vi "microFPGA_laser_duration_addr_10_ctrl.vi"(0 "VISA resource name":refnum<visa-resource-name>, 1 "laser channel":u16(ring)=3 items=["channel No 0", "channel No 1", "channel No 2", "channel No 3", "channel No 4", "channel No 5", "channel No 6"], 2 "write or read":u16(ring) items=["read", "write"], 5 "duration write":u32(slide) max=65535 step=1 scale=0.0..65535.0 scale format="%u us", 11 "error in (no error)":errorcluster) -> (4 "VISA resource name 2":refnum<visa-resource-name>, 6 "duration read":u32(slide) max=65535 step=1 scale=0.0..65535.0 scale format="%u us", 8 "value write confirm":bool, 10 "abort_wrong_input":bool, 15 "error out":errorcluster)   [LabVIEW 2018]
panel:
  out "mode read string answer":string
  out "mode read string":string
  out "mode write string":string
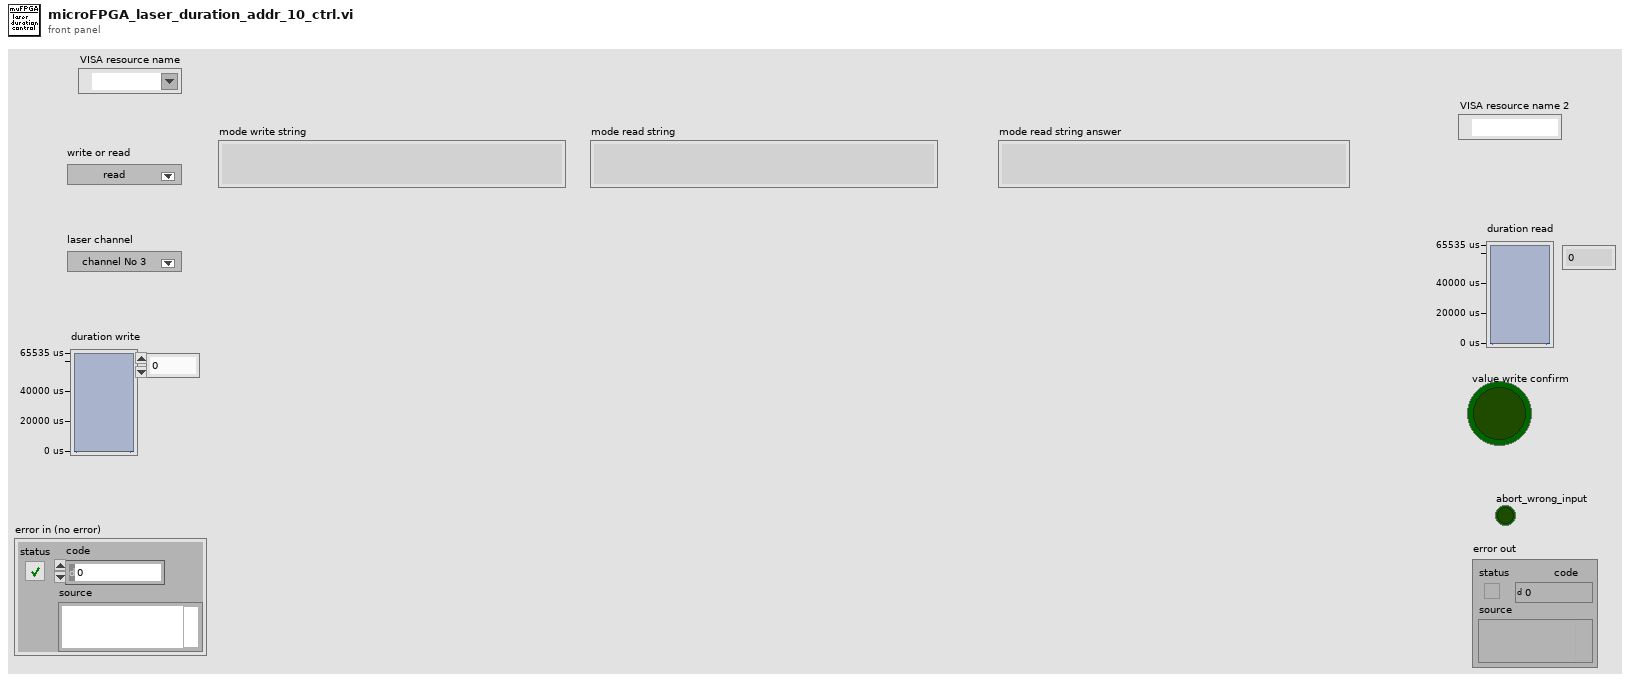
[diagram p1: front panel]
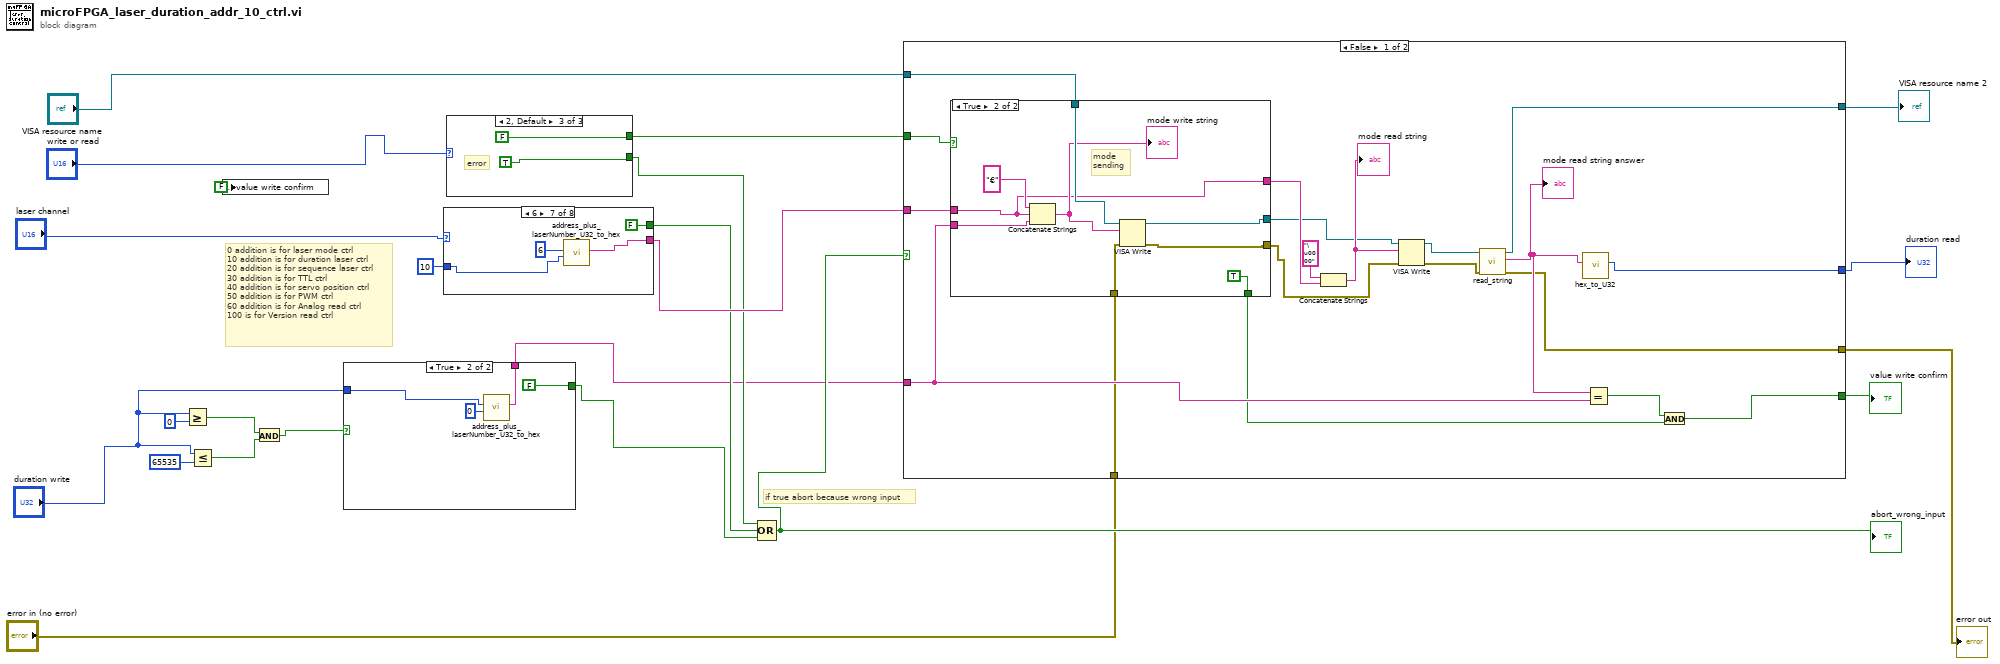
[diagram p0: block diagram]
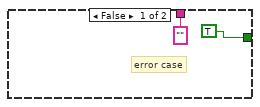
[diagram p2: hidden frame]
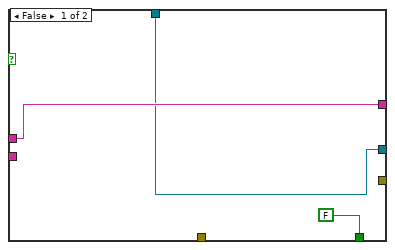
[diagram p3: hidden frame]
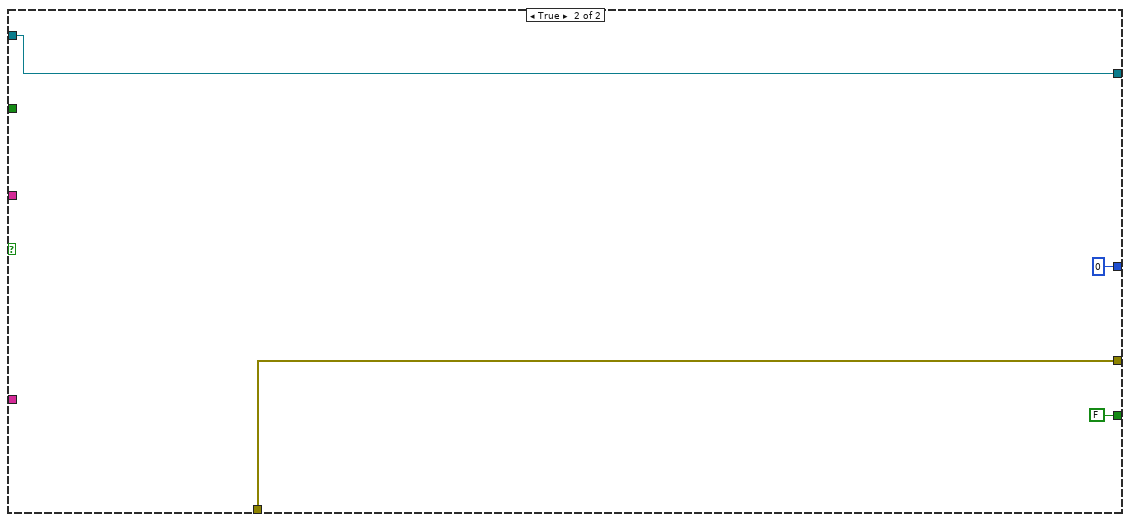
[diagram p4: hidden frame]
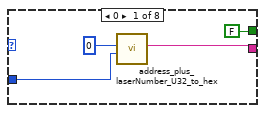
[diagram p5: hidden frame]
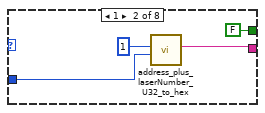
[diagram p6: hidden frame]
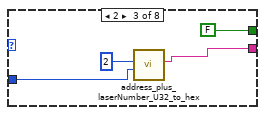
[diagram p7: hidden frame]
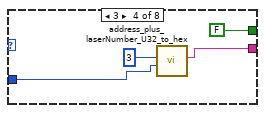
[diagram p8: hidden frame]
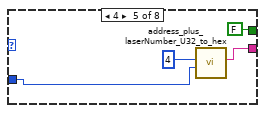
[diagram p9: hidden frame]
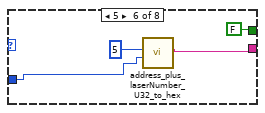
[diagram p10: hidden frame]
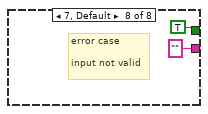
[diagram p11: hidden frame]
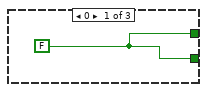
[diagram p12: hidden frame]
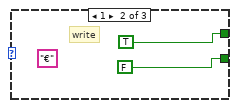
[diagram p13: hidden frame]
diagram:
  # "0 addition is for laser mode ctrl\n10 addition is for duration laser ctrl\n20 addition is for sequence laser ctrl\n30 addition is for TTL ctrl\n40 addition is for servo position ctrl\n50 addition is for PWM ctrl\n60 addition is for Analog read ctrl\n100 is for Version read ctrl"
  # "if true abort because wrong input"
  n1 = Greater Or Equal?(x="duration write", y=u32 0) -> (x >= y?=w7:bool)
  n2 = Less Or Equal?(x="duration write", y=u32 65535) -> (x <= y?=w6:bool)
  n3 = local write "value write confirm"(FALSE ("value confirm")) -> ()
  n4 = And(x=w7, y=w6) -> (x .and. y?=w5:bool)
  n5 = case shown="True" w5 {
    tunnel: "duration write" -> [_ w28]
    tunnel: [TRUE FALSE] -> w4
    tunnel: ["" ("string 5") w26] -> w3
    frame False {
      # "error case"
    }
    frame True {
      n6 = call "address_plus_laserNumber_U32_to_hex.vi"("adress offset"=u32 0, "y 3"=w28) -> ("string 5"=w26:string)  [unwired: 8 in]
    }
  }
  n7 = case shown="6" "laser channel" {
    tunnel: [w31 w35 w39 w43 w47 w51 w55 "" ("string 5")] -> w21
    tunnel: [FALSE FALSE FALSE FALSE FALSE FALSE FALSE TRUE] -> w17
    tunnel: u32 10 ("adress offset") -> [w30 w34 w38 w42 w46 w50 w54 _]
    frame 0 {
      n8 = call "address_plus_laserNumber_U32_to_hex.vi"("adress offset"=w30, "y 3"=u32 0) -> ("string 5"=w31:string)  [unwired: 8 in]
    }
    frame 1 {
      n9 = call "address_plus_laserNumber_U32_to_hex.vi"("adress offset"=w34, "y 3"=u32 1) -> ("string 5"=w35:string)  [unwired: 8 in]
    }
    frame 2 {
      n10 = call "address_plus_laserNumber_U32_to_hex.vi"("adress offset"=w38, "y 3"=u32 2) -> ("string 5"=w39:string)  [unwired: 8 in]
    }
    frame 3 {
      n11 = call "address_plus_laserNumber_U32_to_hex.vi"("adress offset"=w42, "y 3"=u32 3) -> ("string 5"=w43:string)  [unwired: 8 in]
    }
    frame 4 {
      n12 = call "address_plus_laserNumber_U32_to_hex.vi"("adress offset"=w46, "y 3"=u32 4) -> ("string 5"=w47:string)  [unwired: 8 in]
    }
    frame 5 {
      n13 = call "address_plus_laserNumber_U32_to_hex.vi"("adress offset"=w50, "y 3"=u32 5) -> ("string 5"=w51:string)  [unwired: 8 in]
    }
    frame 6 {
      n14 = call "address_plus_laserNumber_U32_to_hex.vi"("adress offset"=w54, "y 3"=u32 6) -> ("string 5"=w55:string)  [unwired: 8 in]
    }
    frame 7, Default {
      # "error case\n\ninput not valid"
    }
  }
  n15 = case shown="2, Default" "write or read" {
    tunnel: [w60 TRUE FALSE] -> w20
    tunnel: [w60 FALSE TRUE] -> w18
    frame 0 {
      w60 = FALSE
    }
    frame 1 {
      (unwired) "€" ("hex")
      # "write"
    }
    frame 2, Default {
      # "error"
    }
  }
  n16 = Compound Arithmetic op=OR(w18, w17, w4) -> (w15:bool)
  "abort_wrong_input" <- w15
  n17 = case shown="False" w15 {
    tunnel: "VISA resource name" -> [w83 w97]
    tunnel: w21 -> [w80 _]
    tunnel: w20 -> [w74 _]
    tunnel: w3 -> [w72 _]
    tunnel: [w71 u32 0 ("U32")] -> w1
    tunnel: [w65 FALSE] -> w16
    tunnel: [w70 w97] -> w14
    tunnel: "error in (no error)" -> [w69 w96]
    tunnel: [w68 w96] -> w12
    frame False {
      n18 = case shown="True" w74 {
        tunnel: w80 -> [w86 w92]
        tunnel: w83 -> [w85 w94]
        tunnel: [w86 w92] -> w81
        tunnel: w72 -> [_ w91]
        tunnel: [w85 w90] -> w76
        tunnel: [_ w89] -> w75
        tunnel: w69 -> [_ w88]
        tunnel: [FALSE TRUE] -> w67
        frame False {
        }
        frame True {
          # "mode \nsending"
          n19 = Concatenate Strings("€" ("string"), w92, w91) -> (w93:string)
          "mode write string" <- w93
          n20 = VISA Write(VISA resource name=w94, write buffer=w93, error in (no error)=w88) -> (VISA resource name out=w90:refnum<visa-resource-name>, error out=w89:errorcluster)  [unwired: 1 out]
        }
      }
      n21 = Concatenate Strings("\u0000" ("string"), w81) -> (w79:string)
      "mode read string" <- w79
      n22 = VISA Write(VISA resource name=w76, write buffer=w79, error in (no error)=w75) -> (VISA resource name out=w78:refnum<visa-resource-name>, error out=w77:errorcluster)  [unwired: 1 out]
      n23 = call "read_string.vi"("error in (no error)"=w77, "VISA resource name 2"=w78) -> ("error out"=w68:errorcluster, "read buffer"=w73:string, "VISA resource name"=w70:refnum<visa-resource-name>)  [unwired: 7 in]
      "mode read string answer" <- w73
      n24 = call "hex_to_U32.vi"("hex"=w73) -> ("U32"=w71:u32)  [unwired: 9 in]
      n25 = Equal?(x=w73, y=w72) -> (x = y?=w66:bool)
      n26 = And(x=w66, y=w67) -> (x .and. y?=w65:bool)
    }
    frame True {
    }
  }
  "value write confirm" <- w16
  "VISA resource name 2" <- w14
  "error out" <- w12
  "duration read" <- w1
